vi "Error Query.vi"(8 "error in (no error)":errorcluster, 11 "VISA resource name":refnum<visa-resource-name>) -> (0 "error out":errorcluster, 1 "Error Message":string, 2 "Error Code":i32, 3 "VISA resource name out":refnum<visa-resource-name>)   [LabVIEW 2014, in "Associated Research SC6540.lvlib"]
doc: "Read an error from the instrument. NOTE: This Operation Is Not Supported By These instruments and the VI will return an Error Query Not Supported Warning Code if the VI is Run."
uses:
  <instrlib>/Associated Research SC6540/Associated Research SC6540.lvlib
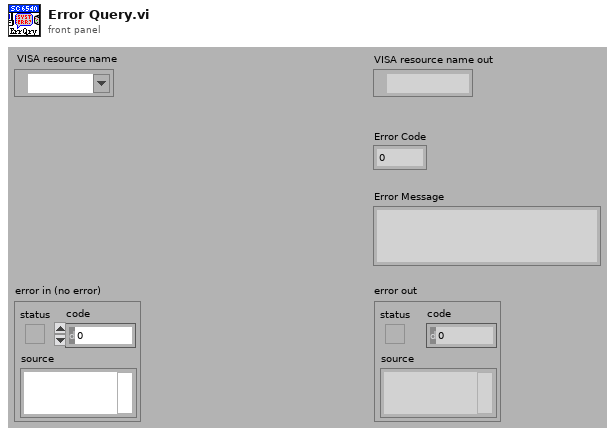
[diagram p1: front panel]
types:
  T1 = cluster{"Operation Complete":bool, "Not Used":bool, "Query Error":bool, "Device Error":bool, "Execution Error":bool, "Command Error":bool, "Not Used":bool, "Power On":bool}
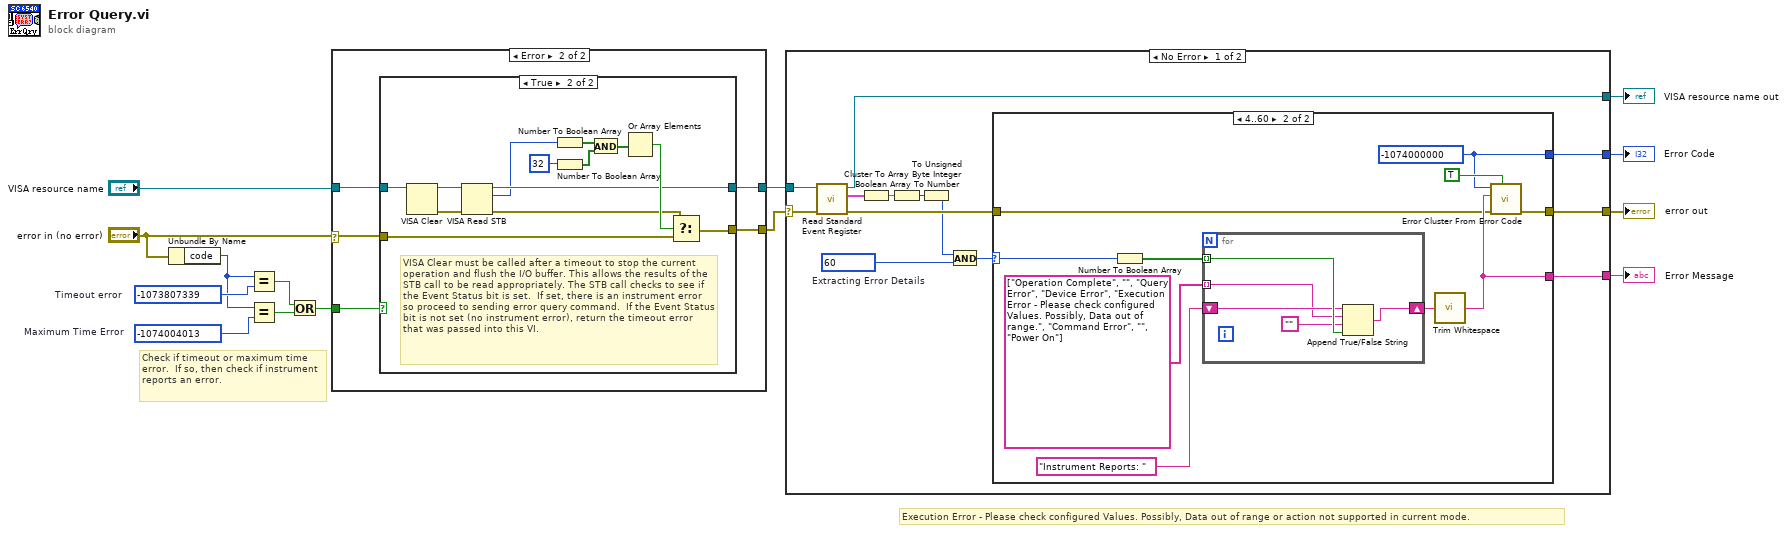
[diagram p0: block diagram]
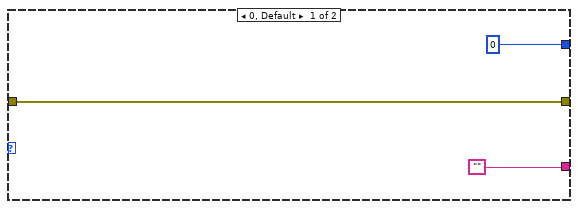
[diagram p4: hidden frame]
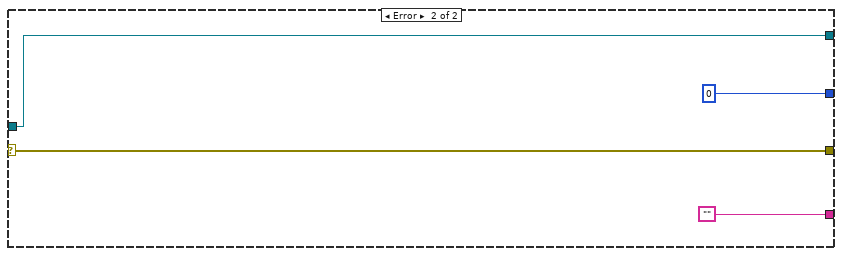
[diagram p5: hidden frame]
diagram:
  w8 = -1074004013  # Maximum Time Error
  w10 = -1073807339  # Timeout error
  # "Check if timeout or maximum time error.  If so, then check if instrument reports an error."
  # "Execution Error - Please check configured Values. Possibly, Data out of range or action not supported in current mode."
  n1 = Unbundle By Name("error in (no error)") -> ("code"=w9:i32)
  n2 = Equal?(x=w9, y=w10) -> (x = y?=w6:bool)
  n3 = Equal?(x=w9, y=w8) -> (x = y?=w7:bool)
  n4 = Or(x=w6, y=w7) -> (x .or. y?=w5:bool)
  n5 = case shown="Error" "error in (no error)" {
    selector: "error in (no error)" -> [w15 w19]
    tunnel: "VISA resource name" -> [w16 w21]
    tunnel: [w16 w20] -> w4
    tunnel: [w15 w18] -> w1
    tunnel: w5 -> [_ w17]
    frame No Error {
    }
    frame Error {
      n6 = case shown="True" w17 {
        tunnel: w21 -> [w23 w29]
        tunnel: [w23 w26] -> w20
        tunnel: w19 -> [w22 w32]
        tunnel: [w22 w31] -> w18
        frame False {
          # "Error code not a timeout, so best to pass on to user."
        }
        frame True {
          # "VISA Clear must be called after a timeout to stop the current operation and flush the I/O buffer. This allows the results of the  STB call to be read appropriately. The STB call checks to see if the Event Status bit is set.  If set, there is an instrument error so proceed to sending error query command.  If the Event Status bit is not set (no instrument error), return the timeout error that was passed into this VI."
          n7 = VISA Clear ("VISA设备清零")(VISA resource name=w29) -> (VISA resource name out=w28:refnum<visa-resource-name>, error out=w27:errorcluster)  [unwired: 1 in]
          n8 = VISA Read STB ("VISA读取STB")(8:w27, 11:w28) -> (0:w25:errorcluster, 2:w24:u16, 3:w26:refnum<visa-resource-name>)
          n9 = Number To Boolean Array(number=w24) -> (Boolean array=w33:bool[])
          n10 = Number To Boolean Array(number=32) -> (Boolean array=w35:bool[])
          n11 = And(x=w33, y=w35) -> (x .and. y?=w34:bool[])
          n12 = Or Array Elements(Boolean array=w34) -> (logical OR=w30:bool)
          n13 = Select(t=w25, s=w30, f=w32) -> (s? t:f=w31:errorcluster)
        }
      }
    }
  }
  n14 = case shown="No Error" w1 {
    selector: w1 -> [w42 w71]
    tunnel: [w41 w70] -> w14
    tunnel: [w49 w71] -> w11
    tunnel: w4 -> [w43 w70]
    tunnel: [w48 "" ("Empty String Constant")] -> w13
    tunnel: [w47 0 ("Code")] -> w12
    frame No Error {
      w46 = u8 60  # Extracting Error Details
      n15 = call <instrlib>:"Read Standard Event Register.vi"("error in (no error)"=w42, "VISA resource name"=w43) -> ("error out"=w39:errorcluster, "Standard Event Register"=w40:T1, "VISA resource name out"=w41:refnum<visa-resource-name>)  [unwired: 7 in]
      n16 = Cluster To Array(cluster=w40) -> (array=w44:bool[])
      n17 = Boolean Array To Number(Boolean array=w44) -> (number=w38:u32)
      n18 = To Unsigned Byte Integer(number=w38) -> (unsigned 8bit integer=w37:u8)
      n19 = And(x=w37, y=w46) -> (x .and. y?=w45:u8)
      n20 = case shown="4..60" w45 {
        selector: w45 -> [_ w57]
        tunnel: [w52 w56] -> w49
        tunnel: w39 -> [w52 w54]
        tunnel: ["" ("Empty String Constant") w55] -> w48
        tunnel: [0 ("Code") w53] -> w47
        frame 0, Default {
        }
        frame 4..60 {
          w53 = -1074000000 ("Code")
          n21 = Number To Boolean Array(number=w57) -> (Boolean array=w61:bool[])
          n22 = for {
            tunnel: w61 -> [w66] mode=indexing
            tunnel: string[] ["Operation Complete", "", "Query Error", "Device Error", "Execution Error - Please check configured Values. Possibly, Data out of range.", "Command Error", "", "Power On"] -> [w64] mode=indexing
            shift-right: [w67] -> w59
            shift-left: "Instrument Reports: " -> [w65]
            n23 = Append True/False String(1:w66, 2:"" ("false string"), 3:w64, 4:w65) -> (0:w67:string)
          }
          n24 = call <vilib>:"Trim Whitespace.vi"("string"=w59) -> ("trimmed string"=w55:string)  [unwired: 1 in]
          n25 = call <vilib>:"Error Cluster From Error Code.vi"("show call chain? (False)"=TRUE, "error in (no error)"=w54, "error message (\"\")"=w55, "error code (0)"=w53) -> ("error out"=w56:errorcluster)  [unwired: 5 in]
        }
      }
    }
    frame Error {
    }
  }
  "Error Message" <- w13
  "error out" <- w11
  "VISA resource name out" <- w14
  "Error Code" <- w12
